vi "mass Cleanup (Library).vi"() -> ()   [LabVIEW 2020]
uses:
  <vilib>/Utility/traverseref.llb/TRef TravTarget.ctl
  <vilib>/Utility/traverseref.llb/VI Scripting - Traverse.lvlib
panel:
  in  "Show FP (F)":bool=TRUE
  out "Slide":u8(slide) scale=0.0..100.0
  out "error":i32
  out "relinked":i32
  in  "Arrange":bool
  in  "FP (T)":bool=TRUE
  in  "Library Path":path=path "C:/Users/Administrator/Desktop/Azdo/emea-aim-664-instrument-driver-1204/src/AIM664LV.lvlib"
  out "error out":errorcluster
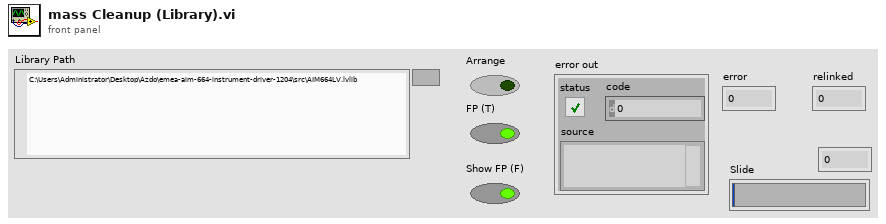
[diagram p1: front panel]
types:
  T1 = typedef "TRef TravTarget.ctl" = enum16{"FP", "BD", "Other"}
  T2 = enum32{"invalid VI type", "Standard VI", "Control VI", "Global VI", "Polymorphic VI", "Configuration VI", "SubSystem", "Facade VI", "Method VI", "Statechart Diagram VI"}
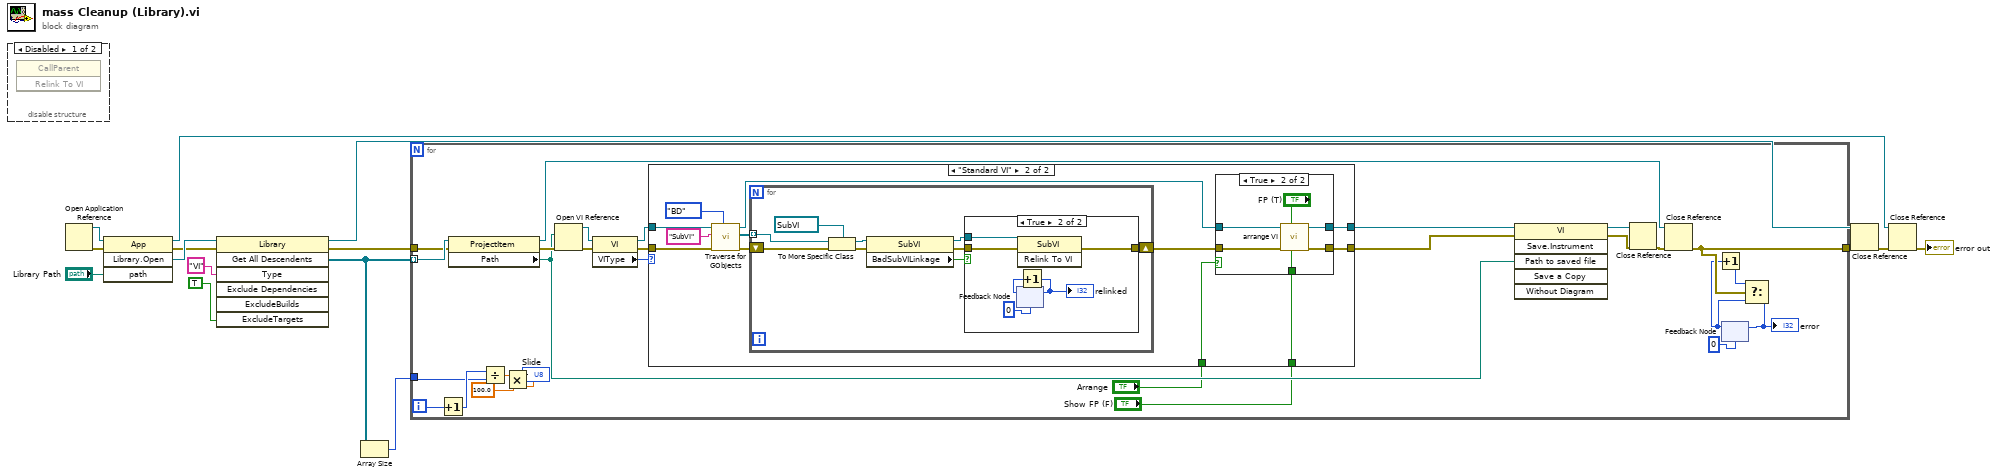
[diagram p0: block diagram]
diagram:
  n1 = disable-structure shown="Disabled" {
    frame Disabled {
      n2 = invoke class="CallParent" method="Relink To VI"() -> ()  [unwired: 3 in, 3 out]
    }
    frame Enabled {
    }
  }
  n3 = Open Application Reference() -> (0:w14:errorcluster, 3:w15:refnum<vi>)  [unwired: 4 in]
  n4 = invoke class="App" method="Library.Open"(reference=w15, error in=w14, "path"="Library Path") -> (reference out=w12:refnum<vi>, error out=w8:errorcluster, "Open Library"=w9:refnum<vi>)  [unwired: 1 in, 1 out]
  n5 = invoke class="Library" method="Get All Descendents"(reference=w9, error in=w8, "Type"="VI", "Exclude Dependencies"=TRUE ("ExcludeDependencies")) -> (reference out=w5:refnum<vi>, error out=w6:errorcluster, "All Descendents"=w2:refnum<vi>[])  [unwired: 3 in, 4 out]
  n6 = Array Size(array=w2) -> (size(s)=w1:i32)
  n7 = for {
    tunnel: w2 -> [w43] mode=indexing
    tunnel: w6 -> [w42]
    tunnel: [w28] -> w4
    tunnel: w1 -> [w23]
    i -> [w31]
    n8 = Increment(x=w31) -> (x+1=w24:i32)
    n9 = property class="ProjectItem"(reference=w43, error in=w42) -> (reference out=w41:refnum<vi>, error out=w40:errorcluster, "Path"=w30:path)
    n10 = Divide(x=w24, y=w23) -> (x/y=w22:dbl)
    n11 = Multiply(x=w22, y=100.0) -> (x*y=→"Slide":dbl)
    n12 = Open VI Reference(vi path=w30, error in (no error)=w40) -> (vi reference=w39:refnum<vi>, error out=w37:errorcluster)  [unwired: 4 in]
    n13 = property class="VI"(reference=w39, error in=w37) -> (reference out=w38:refnum<vi>, error out=w36:errorcluster, "VIType"=w35:T2)
    n14 = case shown="\"Standard VI\"" w35 {
      tunnel: [w45 w46] -> w16
      tunnel: w38 -> [w44 w53]
      tunnel: w36 -> [w45 w52]
      tunnel: "Arrange" -> [_ w51]
      tunnel: "Show FP (F)" -> [_ w48]
      tunnel: [w44 w47] -> w17
      frame "invalid VI type", Default {
      }
      frame "Standard VI" {
        n15 = call <vilib>:"Traverse for GObjects.vi"("Traverse Target"=TRef_TravTarget."BD", "error in (no error)"=w52, "Class Name"="SubVI", "VI Refnum"=w53) -> ("error out"=w55:errorcluster, "References"=w56:refnum<vi>[], "dup VI Refnum"=w49:refnum<vi>)  [unwired: 4 in, 1 out]
        n16 = for {
          tunnel: w56 -> [w72] mode=indexing
          shift-right: [w66] -> w50
          shift-left: w55 -> [w71]
          n17 = To More Specific Class(target class=refnum<vi> refnum ("reference"), reference=w72, error in=w71) -> (specific class reference=w67:refnum<vi>, error out=w74:errorcluster)
          n18 = property class="SubVI"(reference=w67, error in=w74) -> (reference out=w68:refnum<vi>, error out=w69:errorcluster, "BadSubVILinkage"=w70:bool)
          n19 = case shown="True" w70 {
            tunnel: w69 -> [w75 w79]
            tunnel: w68 -> [_ w80]
            tunnel: [w75 w81] -> w66
            frame False {
            }
            frame True {
              n20 = feedback #1(0) -> (w77:i32)
              n21 = invoke class="SubVI" method="Relink To VI"(reference=w80, error in=w79) -> (error out=w81:errorcluster)  [unwired: 1 in, 2 out]
              n22 = Increment(x=w77) -> (x+1=w76:i32)
              "relinked" <- w76
              n23 = feedback-in #1(w76) -> ()
            }
          }
        }
        n24 = case shown="True" w51 {
          tunnel: w50 -> [w58 w65]
          tunnel: [w58 w64] -> w46
          tunnel: w49 -> [w59 w63]
          tunnel: [w59 w62] -> w47
          tunnel: w48 -> [_ w60]
          frame False {
          }
          frame True {
            n25 = call "arrange VI.vi"("Show FP (F)"=w60, "FP (T)"="FP (T)", "error in"=w65, "VI in"=w63) -> ("error out"=w64:errorcluster, "VI out"=w62:refnum<vi>)  [unwired: 6 in]
          }
        }
      }
    }
    n26 = invoke class="VI" method="Save.Instrument"(reference=w17, error in=w16, "Path to saved file"=w30) -> (reference out=w32:refnum<vi>, error out=w33:errorcluster)  [unwired: 3 in, 4 out]
    n27 = Close Reference(reference=w32, error in (no error)=w33) -> (error out=w34:errorcluster)
    n28 = Close Reference(reference=w41, error in (no error)=w34) -> (error out=w28:errorcluster)
    n29 = feedback #2(0) -> (w27:i32)
    n30 = Increment(x=w27) -> (x+1=w26:i32)
    n31 = Select(t=w26, s=w28, f=w27) -> (s? t:f=w25:i32)
    "error" <- w25
    n32 = feedback-in #2(w25) -> ()
  }
  n33 = Close Reference(reference=w5, error in (no error)=w4) -> (error out=w11:errorcluster)
  n34 = Close Reference(reference=w12, error in (no error)=w11) -> (error out=→"error out":errorcluster)
